vi "EnqueueManager (Scalar)__slk_QSM-PC (String).vi"(8 "error in (no error)":errorcluster, 9 "action (back)":enum16{"Back", "Front", "Replace"}(ring), 10 "element":cluster{"State":string, "Data":variant}, 11 "queue in":refnum<queue>) -> (0 "error out":errorcluster)   [LabVIEW 2009, in "QSM-PC (String).lvlib"]
doc: "Sets elements to the different position of queue.\n\n<b>Functions:</b>\nEnqueue to the back of queue\nEnqueue to the front of queue\nReplace the elements of queue"
uses:
  Library/QSM-PC (String).lvlib
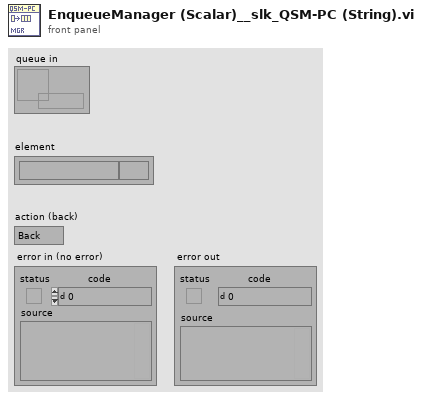
[diagram p1: front panel]
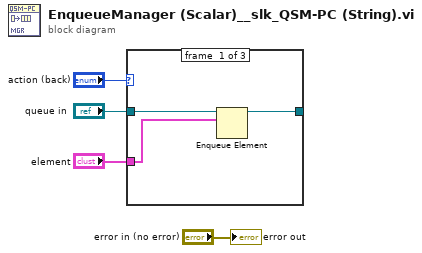
[diagram p0: block diagram]
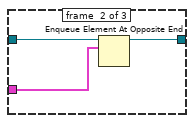
[diagram p2: hidden frame]
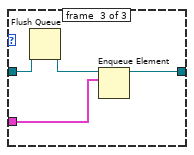
[diagram p3: hidden frame]
diagram:
  n1 = case shown="\"Replace\"" "action (back)" {
    tunnel: "queue in" -> [w7 w10 w12]
    tunnel: "element" -> [w6 w8 w13]
    tunnel: [w5 w9 w14] -> _
    frame #0 {
      n2 = Enqueue Element(queue=w7, element=w6) -> (queue out=w5:refnum<queue>)  [unwired: 1 in, 3 out]
    }
    frame #1 {
      n3 = Enqueue Element At Opposite End(queue=w10, element=w8) -> (queue out=w9:refnum<queue>)  [unwired: 1 in, 3 out]
    }
    frame #2 {
      n4 = Flush Queue(queue=w12) -> (queue out=w11:refnum<queue>)  [unwired: 1 in, 2 out]
      n5 = Enqueue Element(queue=w11, element=w13) -> (queue out=w14:refnum<queue>)  [unwired: 1 in, 3 out]
    }
  }
  "error out" <- "error in (no error)"
